vi "modify menu.vi"() -> ()   [LabVIEW 2013, in "DAQ.lvclass"]
uses:
  DAQ.lvclass
  DAQ.lvclass/DAQ.ctl
  <vilib>/Utility/xml.llb/Write to XML File(string).vi
panel:
  out "Picture":picture
  in  "File Path":path
  in  "Comments":string
  in  "Delete":bool
  in  "Cancel":bool
  in  "Accept":bool
  out "error out":errorcluster
  in  "DAQ.lvclass in":refnum<class "DAQ.lvclass">
  out "DAQ.lvclass out":refnum<class "DAQ.lvclass">
  in  "Measures":string
  in  "Protocols":string
  in  "Analog max":dbl
  in  "Analog min":dbl
  in  "Digital level":dbl
  in  "# of digital I/O":dbl
  in  "Analog outputs":dbl
  in  "Analog inputs":dbl
  in  "Model":string
  in  "Brand":string
  in  "error in (no error)":errorcluster
  # "New / Edit DAQ Model"
  # "Help"
  # "Brand: For example, NI.\n\nModel: For example, SCXI-1000\n\nAnalog inputs/outputs: Enter the max number, even if the model you have has damaged ones.\n\nAnalog min/max: Enter voltage, usually 0 to 5 or -10 to 10.\n\nDigital I/O: Enter the total number of inputs and outputs, damaged or not.\n\nProtocols: Enter the comunications protocols, spaced by commas.\n\nMeasures: Temperature, strain...  enter what is intended and supported.\n\nRefer to the manual for more info."
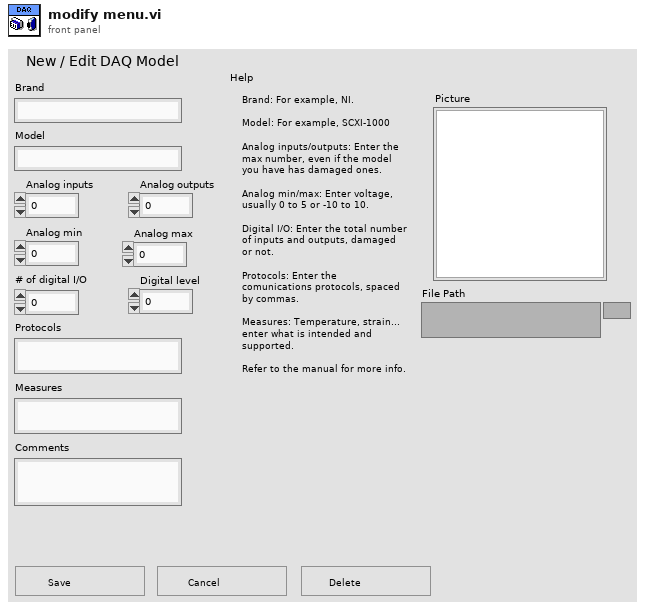
[diagram p1: front panel]
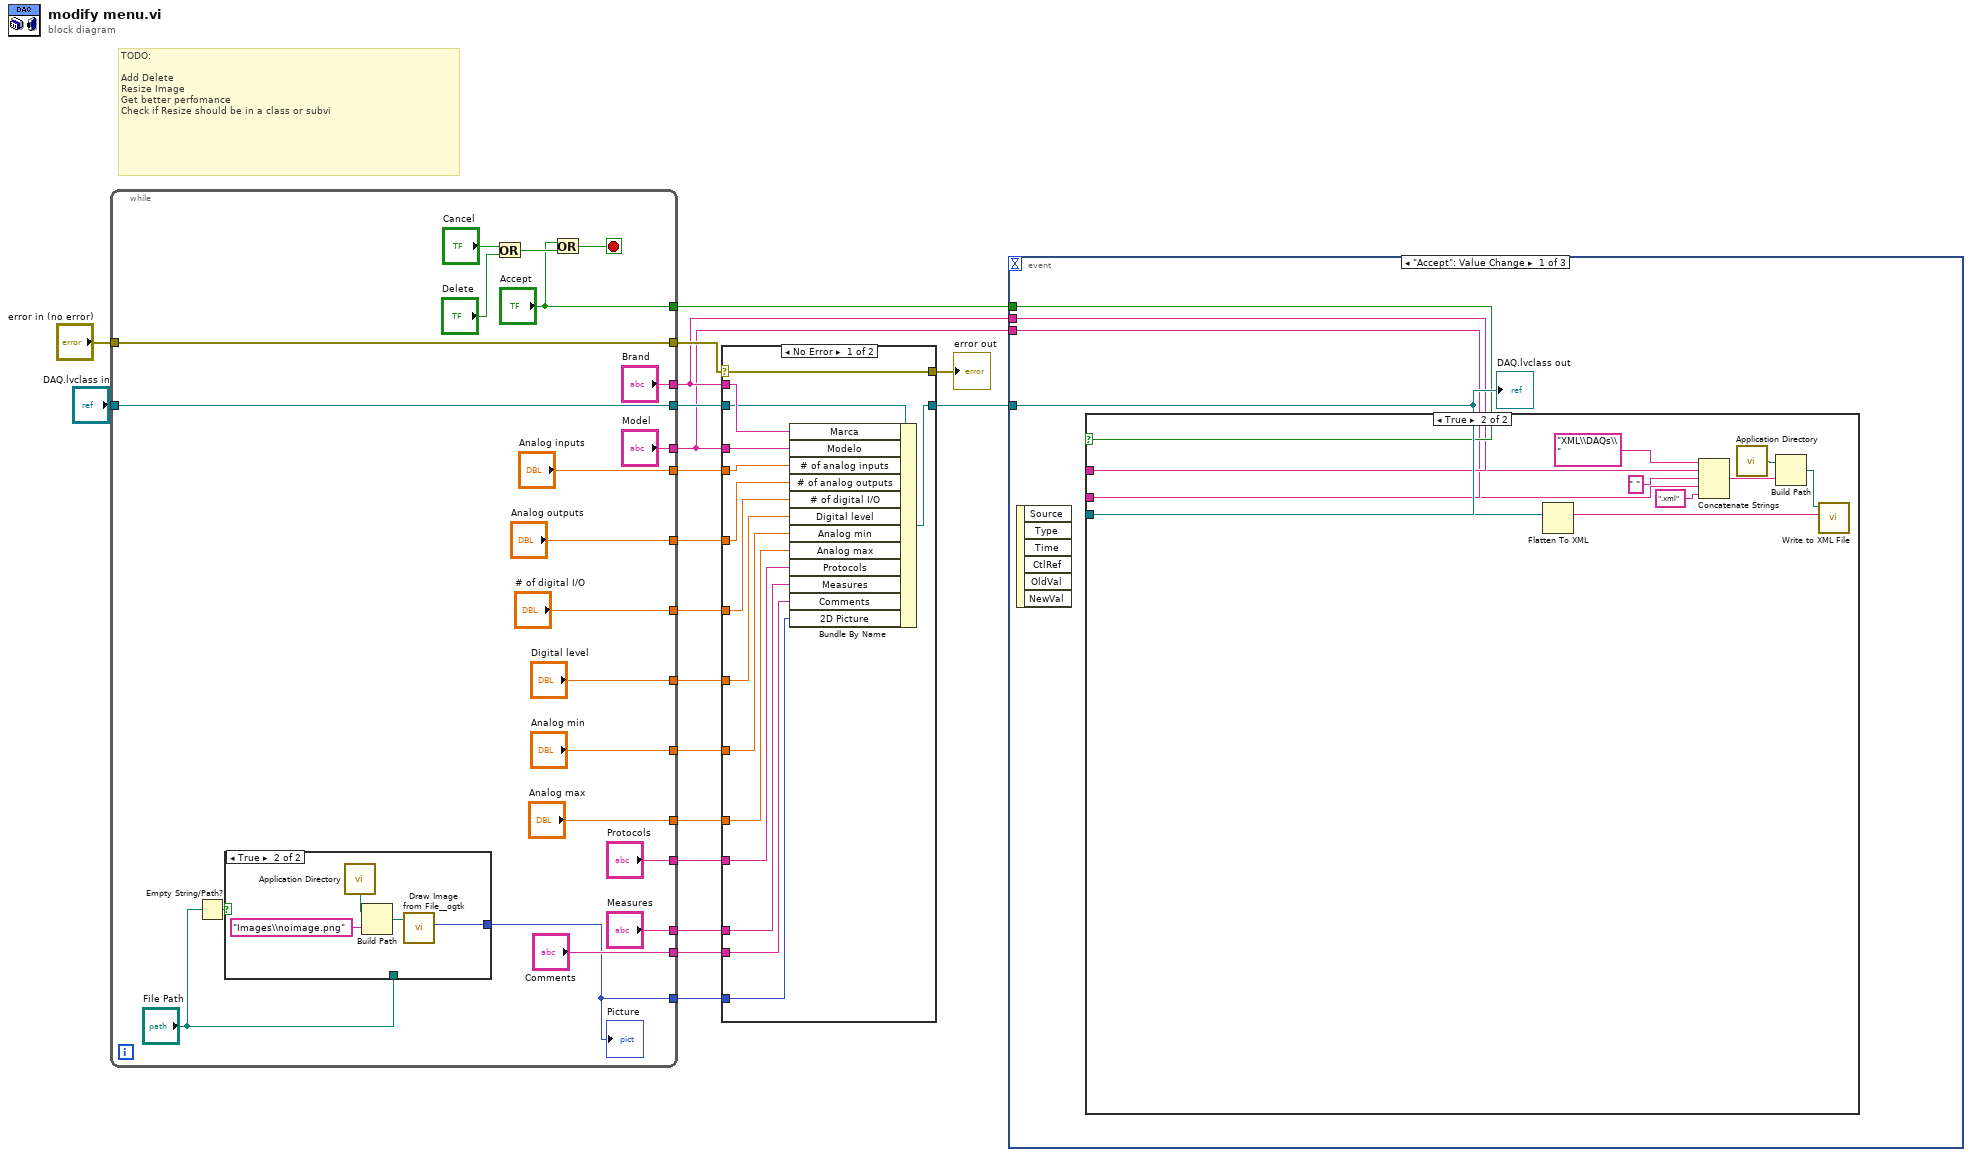
[diagram p0: block diagram]
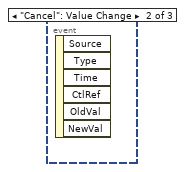
[diagram p4: hidden frame]
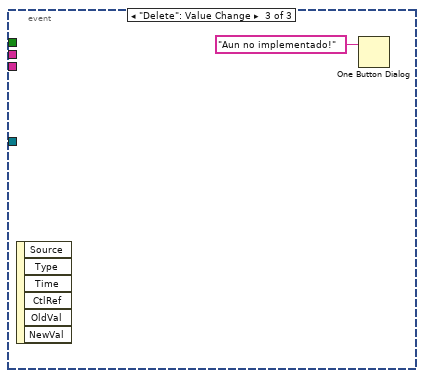
[diagram p5: hidden frame]
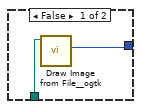
[diagram p6: hidden frame]
diagram:
  # "TODO:\n\nAdd Delete\nResize Image\nGet better perfomance\nCheck if Resize should be in a class or subvi"
  n1 = while {
    tunnel: ["Brand"] -> w3
    tunnel: ["Model"] -> w2
    tunnel: ["Analog inputs"] -> w19
    tunnel: ["Analog outputs"] -> w18
    tunnel: ["# of digital I/O"] -> w17
    tunnel: ["Digital level"] -> w16
    tunnel: ["Analog min"] -> w15
    tunnel: ["Analog max"] -> w14
    tunnel: ["Protocols"] -> w13
    tunnel: ["Measures"] -> w12
    tunnel: ["Comments"] -> w11
    tunnel: [w21] -> w10
    tunnel: [w25] -> w9
    tunnel: "DAQ.lvclass in" -> [w25]
    tunnel: [w24] -> w7
    tunnel: "error in (no error)" -> [w24]
    tunnel: ["Accept"] -> w5
    stop <- w26 stop-if-true
    n2 = Empty String/Path?(string/path="File Path") -> (empty?=w22:bool)
    n3 = case shown="True" w22 {
      tunnel: [w41 w46] -> w21
      tunnel: "File Path" -> [w42 _]
      frame False {
        n4 = call <userlib>:"Draw Image from File__ogtk.vi"("path to image file"=w42) -> ("new picture"=w41:picture)  [unwired: 7 in, 3 out]
      }
      frame True {
        n5 = call <vilib>:"Application Directory.vi"() -> ("Application Directory"=w45:path)
        n6 = Build Path(base path=w45, name or relative path="Images\\noimage.png") -> (appended path=w44:path)
        n7 = call <userlib>:"Draw Image from File__ogtk.vi"("path to image file"=w44) -> ("new picture"=w46:picture)  [unwired: 7 in, 3 out]
      }
    }
    "Picture" <- w21
    n8 = Or(x="Cancel", y="Delete") -> (x .or. y?=w27:bool)
    n9 = Or(x="Accept", y=w27) -> (x .or. y?=w26:bool)
  }
  n10 = case shown="No Error" w7 {
    selector: w7 -> [w60 w63]
    tunnel: [w61 w62] -> w4
    tunnel: [w60 w63] -> w1
    tunnel: w3 -> [w59 _]
    tunnel: w2 -> [w58 _]
    tunnel: w19 -> [w57 _]
    tunnel: w18 -> [w56 _]
    tunnel: w17 -> [w55 _]
    tunnel: w16 -> [w54 _]
    tunnel: w15 -> [w53 _]
    tunnel: w14 -> [w52 _]
    tunnel: w13 -> [w51 _]
    tunnel: w12 -> [w50 _]
    tunnel: w11 -> [w49 _]
    tunnel: w10 -> [w48 _]
    tunnel: w9 -> [w47 w62]
    frame No Error {
      n11 = Bundle By Name(cluster=w47, "Marca"=w59, "Modelo"=w58, "# of analog inputs"=w57, "# of analog outputs"=w56, "# of digital I/O"=w55, "Digital level"=w54, "Analog min"=w53, "Analog max"=w52, "Protocols"=w51, "Measures"=w50, "Comments"=w49, "2D Picture"=w48) -> (w61:refnum<class "DAQ.lvclass">)
    }
    frame Error {
    }
  }
  "error out" <- w1
  n12 = event shown="[0] \"Accept\": Value Change" {
    selector: _ -> [_ _ _]
    dyn-events: _ -> [_ _ _]
    timeout: _ -> [_ _ _]
    tunnel: w4 -> [w67 _ _]
    tunnel: w5 -> [w66 _ _]
    tunnel: w3 -> [w65 _ _]
    tunnel: w2 -> [w64 _ _]
    event "Accept": Value Change {
      n13 = event-data() -> ()  [unwired: 1 in, 6 out]
      n14 = case shown="True" w66 {
        tunnel: w67 -> [_ w73]
        tunnel: w65 -> [_ w71]
        tunnel: w64 -> [_ w69]
        frame False {
        }
        frame True {
          n15 = Flatten To XML(anything=w73) -> (xml string=w72:string)
          n16 = Concatenate Strings("XML\\DAQs\\" ("string"), w71, " " ("string"), w69, ".xml" ("string")) -> (w77:string)
          n17 = call <vilib>:"Application Directory.vi"() -> ("Application Directory"=w75:path)
          n18 = Build Path(base path=w75, name or relative path=w77) -> (appended path=w74:path)
          n19 = call-poly <vilib>:"Write to XML File.vi"("XML Input"=w72, "XML File Path"=w74) -> ()  [unwired: 7 in, 3 out]
        }
      }
      "DAQ.lvclass out" <- w67
    }
    event "Cancel": Value Change {
      n20 = event-data() -> ()  [unwired: 1 in, 6 out]
    }
    event "Delete": Value Change {
      n21 = event-data() -> ()  [unwired: 1 in, 6 out]
      n22 = One Button Dialog(message="Aun no implementado!") -> ()  [unwired: 1 in, 1 out]
    }
  }
